vi "RandomizeArray.vi"   [LabVIEW 2013]
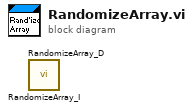
[diagram p0: block diagram]
diagram:
  n1 = call "RandomizeArray_I.vi"() -> ()  [unwired: 10 in, 2 out]
  n2 = call "RandomizeArray_D.vi"() -> ()  [unwired: 10 in, 2 out]
